vi "sub_plot_all_channels.vi"(0 "Is first?":bool=TRUE, 1 "Front_panel_refs":T1, 7 "Plot cluster":T2, 11 "Cluster":cluster{dbl[], dbl[], dbl[]}, 12 "Custom channel":i32, 13 "Total current":dbl, 14 "Data":dbl) -> (8 "Plot cluster out":T2, 15 "Cluster out":cluster{dbl[], dbl[], dbl[]})   [LabVIEW 2016]
doc: "Plots in-time data measured per pad."
uses:
  refs_front_panel.ctl
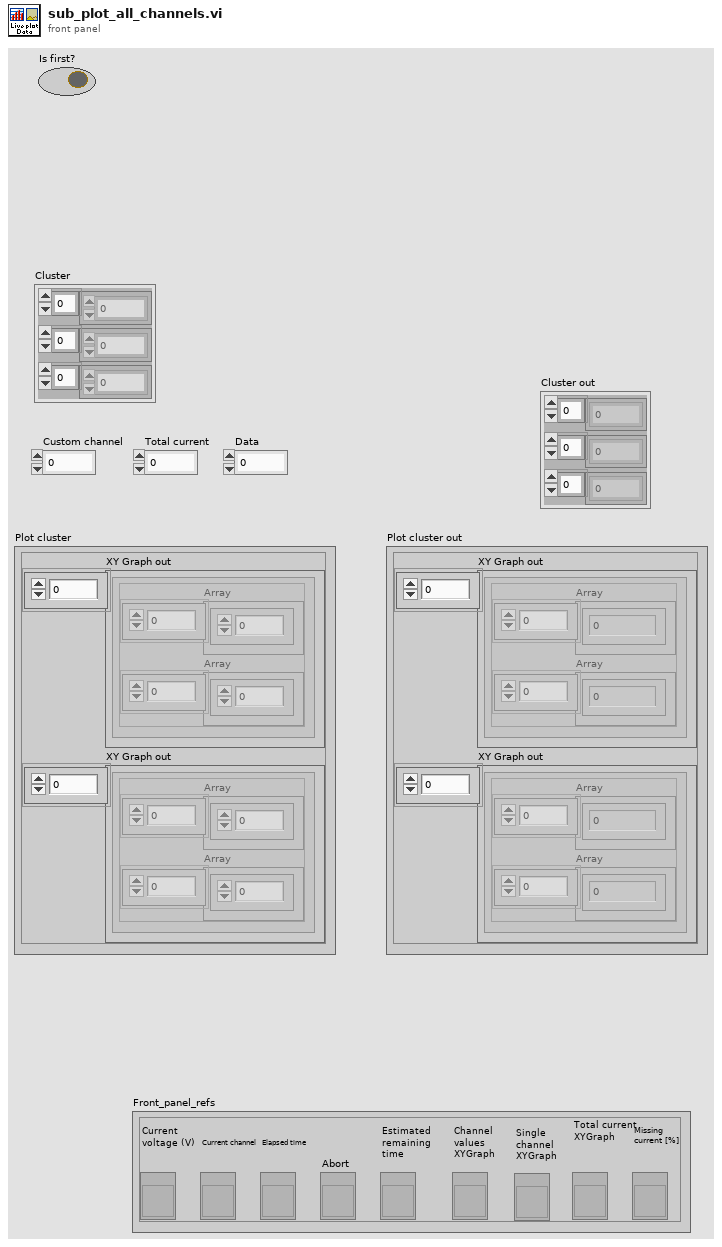
[diagram p1: front panel]
types:
  T1 = typedef "refs_front_panel.ctl" = cluster{"Current voltage (V)":refnum<vi>, "Elapsed time":refnum<vi>, "Current channel":refnum<vi>, "Abort":refnum<vi>, "Estimated remaining time":refnum<vi>, "Channel values XYGraph":refnum<vi>, "Single channel XYGraph":refnum<vi>, "Total current XYGraph":refnum<vi>, "Missing\ncurrent [%]":refnum<vi>}
  T2 = cluster{"XY Graph out":cluster{"Array":dbl[], "Array":dbl[]}[], "XY Graph out":cluster{"Array":dbl[], "Array":dbl[]}[]}
  T3 = cluster{"Y array out":dbl[], "X array out":dbl[], "Y array out":dbl[]}
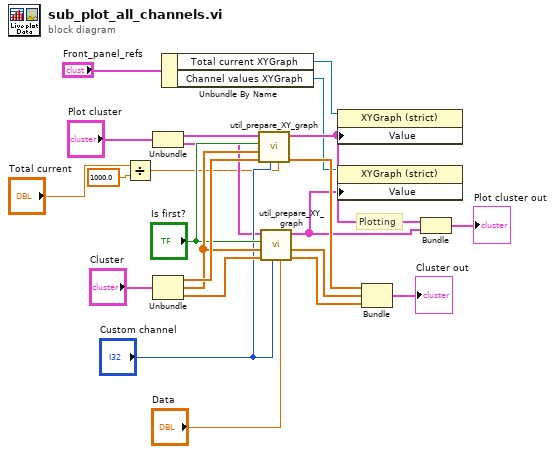
[diagram p0: block diagram]
diagram:
  # "Plotting"
  n1 = Divide(x="Total current", y=1000.0) -> (x/y=w4:dbl)
  n2 = Unbundle("Plot cluster") -> ("XY Graph out"=w8:cluster{"Array":dbl[], "Array":dbl[]}[], "XY Graph out"=w7:cluster{"Array":dbl[], "Array":dbl[]}[])
  n3 = Unbundle("Cluster") -> (w23:dbl[], w22:dbl[], w21:dbl[])
  n4 = Unbundle By Name("Front_panel_refs") -> ("Total current XYGraph"=w2:refnum<vi>, "Channel values XYGraph"=w1:refnum<vi>)
  n5 = call "util_prepare_XY_graph.vi"("Y"=w4, "X"="Custom channel", "Y array"=w23, "X array"=w22, "IsFirst"="Is first?", "XY Graph in"=w8) -> ("Y array out"=w18:dbl[], "XY Graph out"=w12:cluster{"Array":dbl[], "Array":dbl[]}[])  [unwired: 3 in, 1 out]
  n6 = call "util_prepare_XY_graph.vi"("Y"="Data", "X"="Custom channel", "Y array"=w21, "X array"=w22, "IsFirst"="Is first?", "XY Graph in"=w7) -> ("Y array out"=w20:dbl[], "X array out"=w19:dbl[], "XY Graph out"=w11:cluster{"Array":dbl[], "Array":dbl[]}[])  [unwired: 3 in]
  n7 = property class="XYGraph (strict)"(reference=w2, "Value"=w12) -> ()  [unwired: 1 in, 2 out]
  n8 = property class="XYGraph (strict)"(reference=w1, "Value"=w11) -> ()  [unwired: 1 in, 2 out]
  n9 = Bundle("Y array out"=w18, "X array out"=w19, "Y array out"=w20) -> (→"Cluster out":T3)  [unwired: 1 in]
  n10 = Bundle("XY Graph out"=w12, "XY Graph out"=w11) -> (→"Plot cluster out":T2)  [unwired: 1 in]
